vi "3-lorentzian-parameters - manage.vi"(0 "ζ":dbl(slide)=0.00391493831404709 min=0.0 max=0.3 step=1e-06 scale=1e-05..1000.0 scale format="%#_3p", 1 "T1":dbl(slide)=0.009762017848695768 min=0.0 max=0.3 step=1e-06 scale=0.0001..10.0 scale format="%#_3p", 2 "τS":dbl(slide)=0.13437466196040418 min=0.0 max=0.3 step=1e-06 scale=0.0001..10.0 scale format="%#_3p", 3 "τN":dbl(slide)=4.235643214853134e-05 min=0.0 max=0.3 step=1e-06 scale=1e-06..10.0 scale format="%#_3p", 4 "τC":dbl(slide)=0.013647490503661961 min=0.0 max=0.3 step=1e-06 scale=0.0001..10.0 scale format="%#_3p", 5 "κ0":dbl(slide)=1.0234079529926423e-07 min=0.0 max=0.3 step=1e-12 scale=1e-10..1e-06 scale format="%#_3p", 7 "parameter array":dbl[](array[numeric]), 8 "parameters":T1) -> (13 "parameter array OUT":dbl[](array[numeric]), 14 "ζ OUT":dbl(slide)=0.00391493831404709 min=0.0 max=0.3 step=1e-06 scale=1e-05..1000.0 scale format="%#_3p", 15 "T1 OUT":dbl(slide)=0.009762017848695768 min=0.0 max=0.3 step=1e-06 scale=0.0001..10.0 scale format="%#_3p", 16 "τS  OUT":dbl(slide)=0.13437466196040418 min=0.0 max=0.3 step=1e-06 scale=0.0001..10.0 scale format="%#_3p", 17 "τN  OUT":dbl(slide)=4.235643214853134e-05 min=0.0 max=0.3 step=1e-06 scale=1e-06..10.0 scale format="%#_3p", 18 "τC  OUT":dbl(slide)=0.013647490503661961 min=0.0 max=0.3 step=1e-06 scale=0.0001..10.0 scale format="%#_3p", 19 "κ0  OUT":dbl(slide)=1.0234079529926423e-07 min=0.0 max=0.3 step=1e-12 scale=1e-10..1e-06 scale format="%#_3p")   [LabVIEW 2020]
uses:
  3-lorentzian-parameters -- action.ctl
  3-lorentzian-parameters.ctl
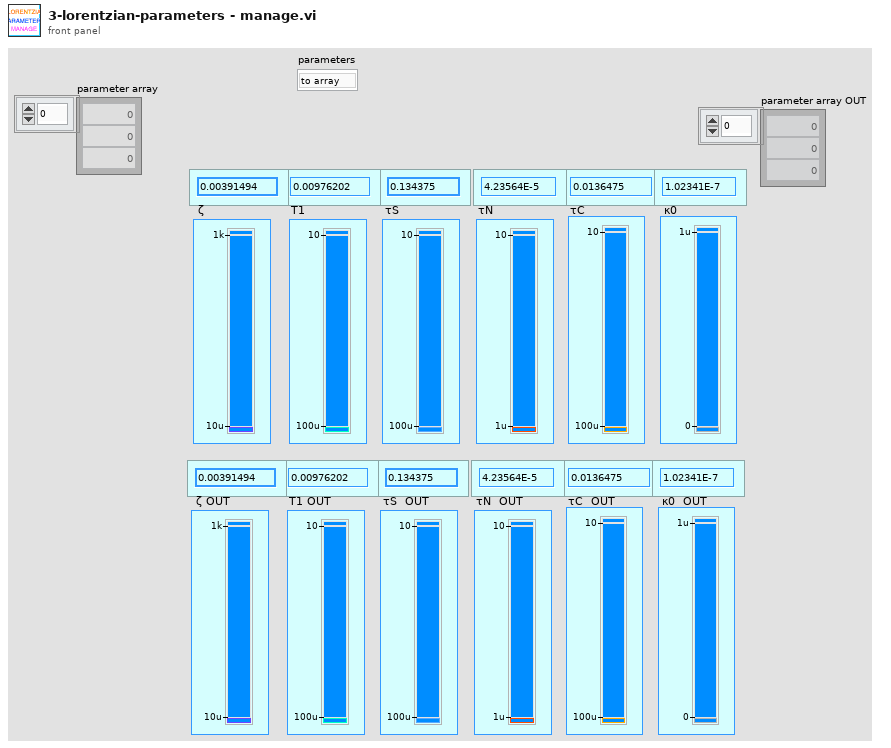
[diagram p1: front panel]
types:
  T1 = typedef "3-lorentzian-parameters -- action.ctl" = enum16{"to array", "to parameters"}
  T2 = typedef "3-lorentzian-parameters.ctl" = enum16{"ζ", "τ1", "τS", "τN", "τC", "κ0", "m1", "m2", "m3", "T (K)", "B (T)", "θ (deg)", "side (S|R)", "change (B|T)"}
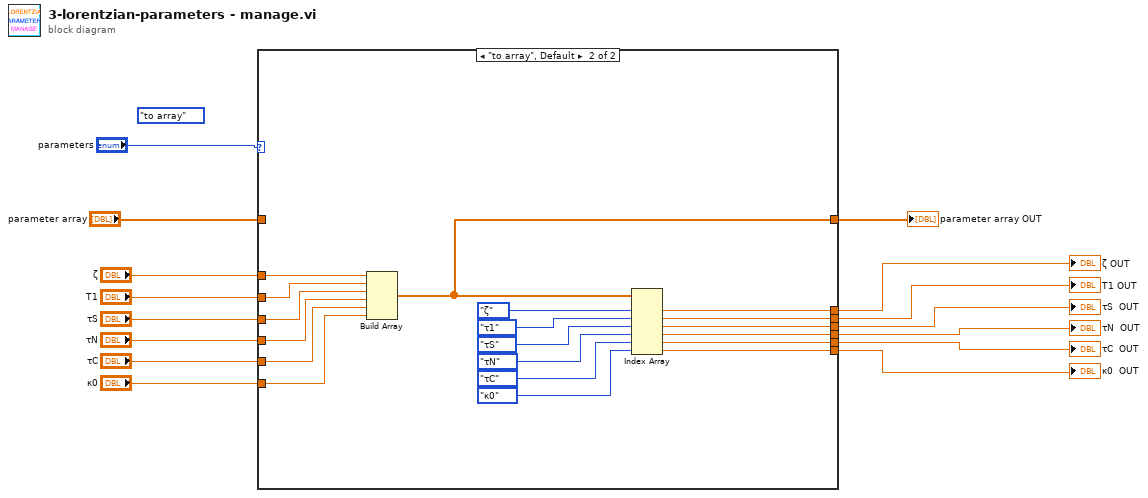
[diagram p0: block diagram]
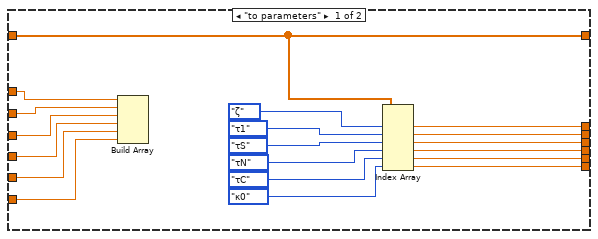
[diagram p2: hidden frame]
diagram:
  (unwired) 3-lorentzian-parameters_--_action."to array" ("parameters")
  n1 = case shown="\"to array\", Default" "parameters" {
    tunnel: [w28 w47] -> w15
    tunnel: [w27 w46] -> w14
    tunnel: [w26 w45] -> w13
    tunnel: [w25 w44] -> w12
    tunnel: [w24 w43] -> w11
    tunnel: [w23 w42] -> w10
    tunnel: "ζ" -> [w22 w41]
    tunnel: "T1" -> [w21 w40]
    tunnel: "τS" -> [w20 w39]
    tunnel: "τN" -> [w19 w38]
    tunnel: "τC" -> [w18 w37]
    tunnel: "κ0" -> [w17 w36]
    tunnel: "parameter array" -> [w16 _]
    tunnel: [w16 w35] -> w1
    frame "to parameters" {
      n2 = Build Array(w22, w21, w20, w19, w18, w17) -> ()  [unwired: 1 out]
      n3 = Index Array(array=w16, index #1=3-lorentzian-parameters."ζ" ("Plost: sweep window"), index #2=3-lorentzian-parameters."τ1" ("Plost: sweep window"), index #3=3-lorentzian-parameters."τS" ("Plost: sweep window"), index #4=3-lorentzian-parameters."τN" ("Plost: sweep window"), index #5=3-lorentzian-parameters."τC" ("Plost: sweep window"), index #6=3-lorentzian-parameters."κ0" ("Plost: sweep window")) -> (element #1=w28:dbl, element #2=w27:dbl, element #3=w26:dbl, element #4=w25:dbl, element #5=w24:dbl, element #6=w23:dbl)
    }
    frame "to array", Default {
      n4 = Build Array(w41, w40, w39, w38, w37, w36) -> (w35:dbl[])
      n5 = Index Array(array=w35, index #1=3-lorentzian-parameters."ζ" ("Plost: sweep window"), index #2=3-lorentzian-parameters."τ1" ("Plost: sweep window"), index #3=3-lorentzian-parameters."τS" ("Plost: sweep window"), index #4=3-lorentzian-parameters."τN" ("Plost: sweep window"), index #5=3-lorentzian-parameters."τC" ("Plost: sweep window"), index #6=3-lorentzian-parameters."κ0" ("Plost: sweep window")) -> (element #1=w47:dbl, element #2=w46:dbl, element #3=w45:dbl, element #4=w44:dbl, element #5=w43:dbl, element #6=w42:dbl)
    }
  }
  "τS  OUT" <- w13
  "τC  OUT" <- w11
  "T1 OUT" <- w14
  "τN  OUT" <- w12
  "ζ OUT" <- w15
  "κ0  OUT" <- w10
  "parameter array OUT" <- w1
